vi "Close Instrument.vi"(7 "Go Local (\"@LOC\")":bool, 8 "error in (no error)":errorcluster, 11 "Instrument in":refnum<class "Instrument.lvclass">) -> (0 "error out":errorcluster, 3 "Instrument out":refnum<class "Instrument.lvclass">)   [LabVIEW 2020, in "Instrument.lvclass"]
uses:
  Instrument.lvclass
  Instrument.lvclass/Instrument.ctl
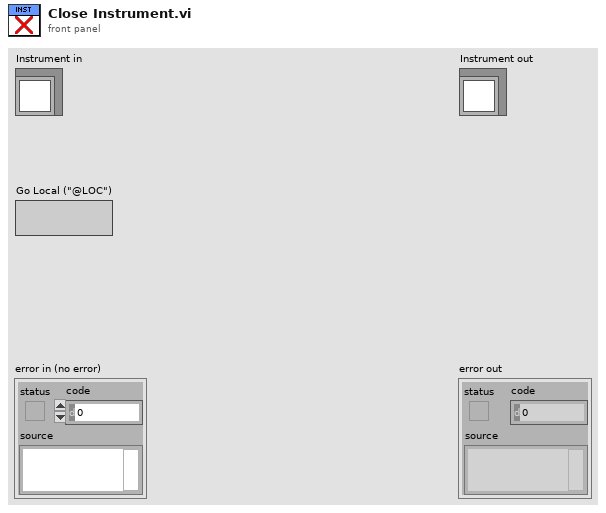
[diagram p1: front panel]
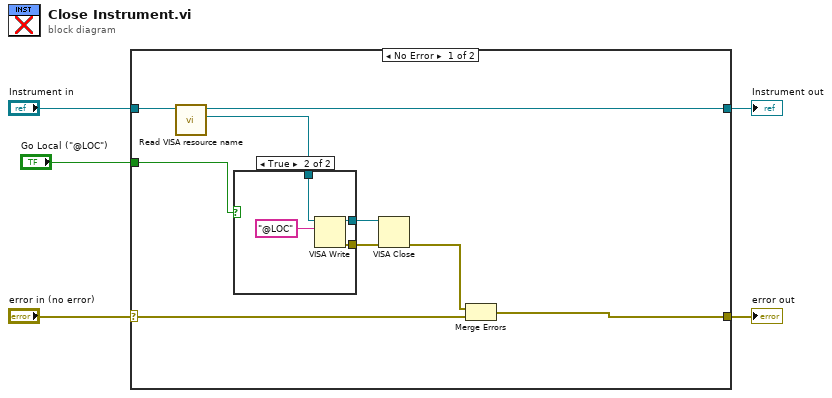
[diagram p0: block diagram]
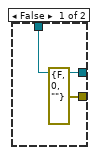
[diagram p2: hidden frame]
diagram:
  n1 = case shown="No Error" "error in (no error)" {
    selector: "error in (no error)" -> [w8 w22]
    tunnel: [w6 w22] -> w4
    tunnel: [w12 w21] -> w2
    tunnel: "Instrument in" -> [w14 w21]
    tunnel: "Go Local (\"@LOC\")" -> [w9 _]
    frame No Error {
      n2 = call "Read VISA resource name.vi"("Instrument in"=w14) -> ("VISA resource name"=w13:refnum<visa-resource-name>, "Instrument out"=w12:refnum<class "Instrument.lvclass">)  [unwired: 9 in]
      n3 = case shown="True" w9 {
        tunnel: w13 -> [w16 w20]
        tunnel: [errorcluster {"status"=FALSE, "code"=0, "source"=""} ("error out") w18] -> w11
        tunnel: [w16 w17] -> w10
        frame False {
        }
        frame True {
          n4 = VISA Write(VISA resource name=w20, write buffer="@LOC") -> (VISA resource name out=w17:refnum<visa-resource-name>, error out=w18:errorcluster)  [unwired: 1 in, 1 out]
        }
      }
      n5 = VISA Close(VISA resource name=w10, error in (no error)=w11) -> (error out=w7:errorcluster)
      n6 = Merge Errors(w7, w8) -> (w6:errorcluster)
    }
    frame Error {
    }
  }
  "error out" <- w4
  "Instrument out" <- w2
